vi "Tree.vi"   [LabVIEW 2016, in "LV-Data.S3.lvclass"]
uses:
  LV-Data.S3.lvclass
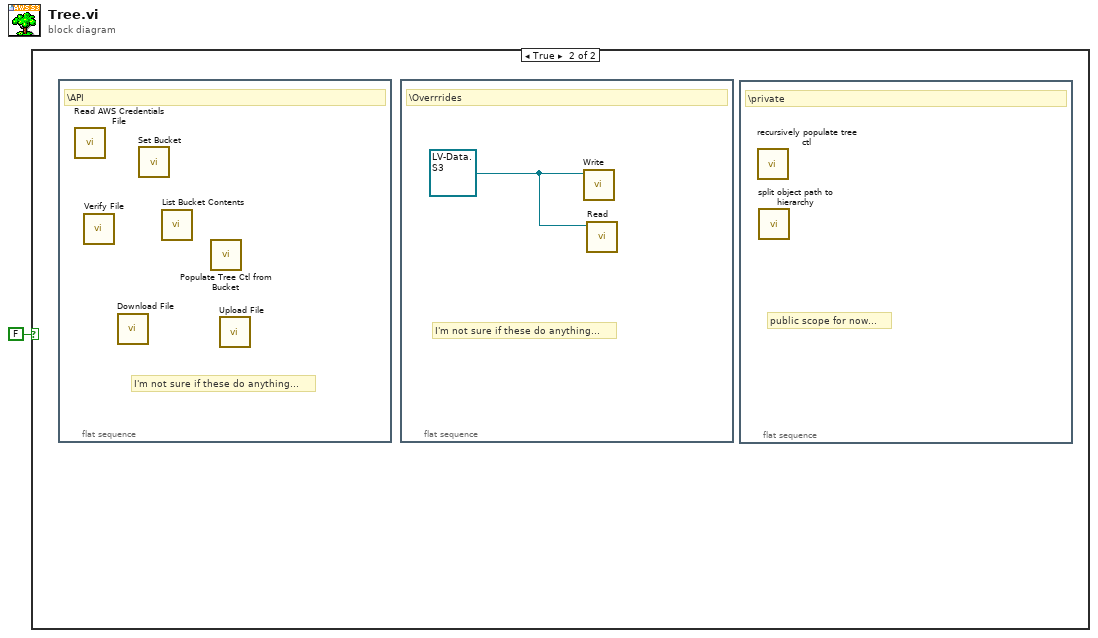
[diagram p0: block diagram]
diagram:
  n1 = case shown="True" FALSE {
    frame False {
    }
    frame True {
      n2 = flat-sequence {
        frame #0 {
          # "I'm not sure if these do anything..."
          # "\\API"
          n3 = call "Read AWS Credentials File.vi"() -> ()  [unwired: 9 in, 3 out]
          n4 = call "Verify File.vi"() -> ()  [unwired: 9 in, 3 out]
          n5 = call "Download File.vi"() -> ()  [unwired: 9 in, 3 out]
          n6 = call "Set Bucket.vi"() -> ()  [unwired: 10 in, 2 out]
          n7 = call "List Bucket Contents.vi"() -> ()  [unwired: 8 in, 4 out]
          n8 = call "Populate Tree Ctl from Bucket.vi"() -> ()  [unwired: 7 in, 5 out]
          n9 = call "Upload File.vi"() -> ()  [unwired: 10 in, 2 out]
        }
      }
      n10 = flat-sequence {
        frame #0 {
          w2 = refnum<class "LV-Data.S3.lvclass"> refnum ("Data.S3")
          # "I'm not sure if these do anything..."
          # "\\Overrrides"
          n11 = call-dynamic "Write.vi"("Data.S3"=w2) -> ()  [unwired: 8 in, 3 out]
          n12 = call-dynamic "Read.vi"("Data.S3"=w2) -> ()  [unwired: 6 in, 5 out]
        }
      }
      n13 = flat-sequence {
        frame #0 {
          # "public scope for now..."
          # "\\private"
          n14 = call "recursively populate tree ctl.vi"() -> ()  [unwired: 10 in, 2 out]
          n15 = call "split object path to hierarchy.vi"() -> ()  [unwired: 8 in, 4 out]
        }
      }
    }
  }
